vi "BC Async HP Data - SA.vi"(8 "error in (no error)":errorcluster, 11 "Bus Controller in":refnum<class "Bus Controller.lvclass">) -> (0 "error out":errorcluster, 3 "Bus Controller out":refnum<class "Bus Controller.lvclass">)   [LabVIEW 2020, in "Unit Tests.lvlib" / "Bus Controller.lvclass"]
uses:
  Bus Controller.lvclass
  Frames & Messages/TypeDefs/Async Message Config.ctl
  Frames & Messages/TypeDefs/Command Config.ctl
  Frames & Messages/TypeDefs/Command Type.ctl
  Frames & Messages/TypeDefs/Command Terminal Address.ctl
  Frames & Messages/TypeDefs/Command SubAddress.ctl
  Frames & Messages/TypeDefs/Command Word Count.ctl
  Frames & Messages/TypeDefs/Message Control.ctl
  Frames & Messages/TypeDefs/Simplified Parameter Data Table.ctl
  Frames & Messages/TypeDefs/Scaling Information.ctl
  Bus Controller.lvclass/Bus Controller.ctl
  1553 Session/1553 Session.lvclass/1553 Session.ctl
  Bus Controller/Bus Controller.lvclass
  1553 Component/1553 Component.lvclass/1553 Component.ctl
  <vilib>/addons/_JKI Toolkits/Caraya/classes/Assert/Assert True.vi
  1553 Component/1553 Component.lvclass
  1553 SubComponent/1553 SubComponent.lvclass
  Dependencies/FPGA Interface/FPGA Interface.lvclass
  <vilib>/addons/_JKI Toolkits/Caraya/classes/Test/Test.lvclass
  Frames & Messages/Async Message/Async Message.lvclass
  BCI-1553 API.lvlib
  1553 Session/1553 Session.lvclass
  <vilib>/addons/_JKI Toolkits/Caraya/classes/Assert/Assert.lvclass
panel:
  out "Data":u16[](array[numeric]) format="%04x"
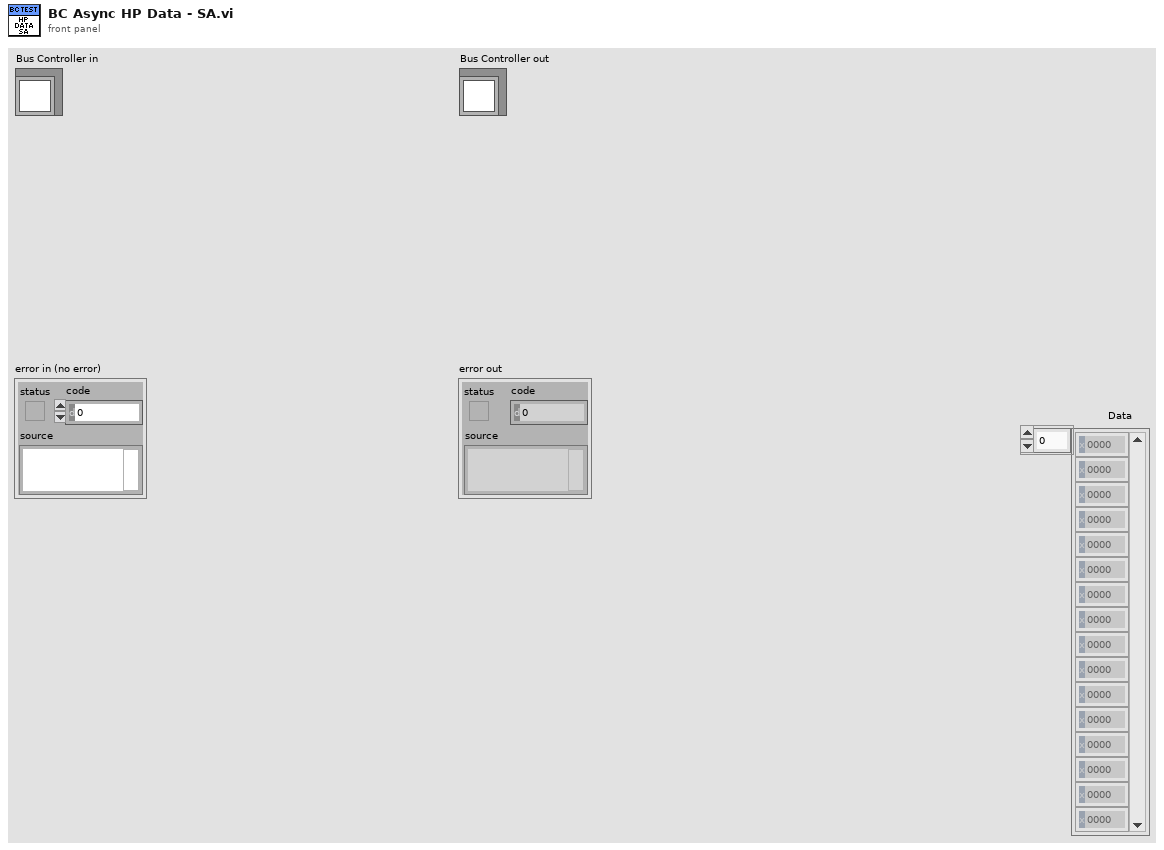
[diagram p1: front panel]
types:
  T1 = typedef "BCI-1553 API.lvlib/Command Word Count.ctl" = enum16{"1", "2", "3", "4", "5", "6", "7", "8", "9", "10", "11", "12", "13", "14", "15", "16", "17", "18", "19", "20", "21", "22", "23", "24", "25", "26", "27", "28", "29", "30", "31", "32"}
  T2 = typedef "BCI-1553 API.lvlib/Command SubAddress.ctl" = enum16{"Mode Code", "1", "2", "3", "4", "5", "6", "7", "8", "9", "10", "11", "12", "13", "14", "15", "16", "17", "18", "19", "20", "21", "22", "23", "24", "25", "26", "27", "28", "29", "30"}
  T3 = typedef "BCI-1553 API.lvlib/Command Terminal Address.ctl" = enum16{"0", "1", "2", "3", "4", "5", "6", "7", "8", "9", "10", "11", "12", "13", "14", "15", "16", "17", "18", "19", "20", "21", "22", "23", "24", "25", "26", "27", "28", "29", "30", "Broadcast"}
  T4 = typedef "BCI-1553 API.lvlib/Command Type.ctl" = enum16{"Transmit", "Receive"}
  T5 = typedef "BCI-1553 API.lvlib/Simplified Parameter Data Table.ctl" = cluster{"Parameter Name":string, "Base Word":u16, "Scaling Info":T6}
  T6 = typedef "BCI-1553 API.lvlib/Scaling Information.ctl" = cluster{"Bit Offset":i32, "Bit Count":i32, "LSB Resolution":dbl, "2's Complement":bool, "Big Endian":bool, "Sign Bit":bool}
  T7 = typedef "BCI-1553 API.lvlib/Command Config.ctl" = cluster{"Command Type":T4, "Terminal Address":T3, "SubAddress":T2, "Word Count\\Mode Code":T1, "Command Data":u16[]}
  T8 = typedef "BCI-1553 API.lvlib/Async Message Config.ctl" = cluster{"Group":i32, "High Priority":bool, "Time to Next Msg (100 us)":u16, "Command Config":T7, "Message Control":T9}
  T9 = typedef "BCI-1553 API.lvlib/Message Control.ctl" = cluster{"MC17 Time Sync":bool, "Error Mask":bool, "Service Request Mask":bool, "Busy Mask":bool, "SubSystem Flag Mask":bool, "Terminal Flag Mask":bool, "Reserved Mask":bool, "Retry":bool, "Bus A / !Bus B":bool, "Self-Test Loopback":bool, "Broadcast Mask":bool, "EoM Interrupt":bool, "Mode Code Format":bool, "Broadcast Format":bool, "RT-RT Format":bool}
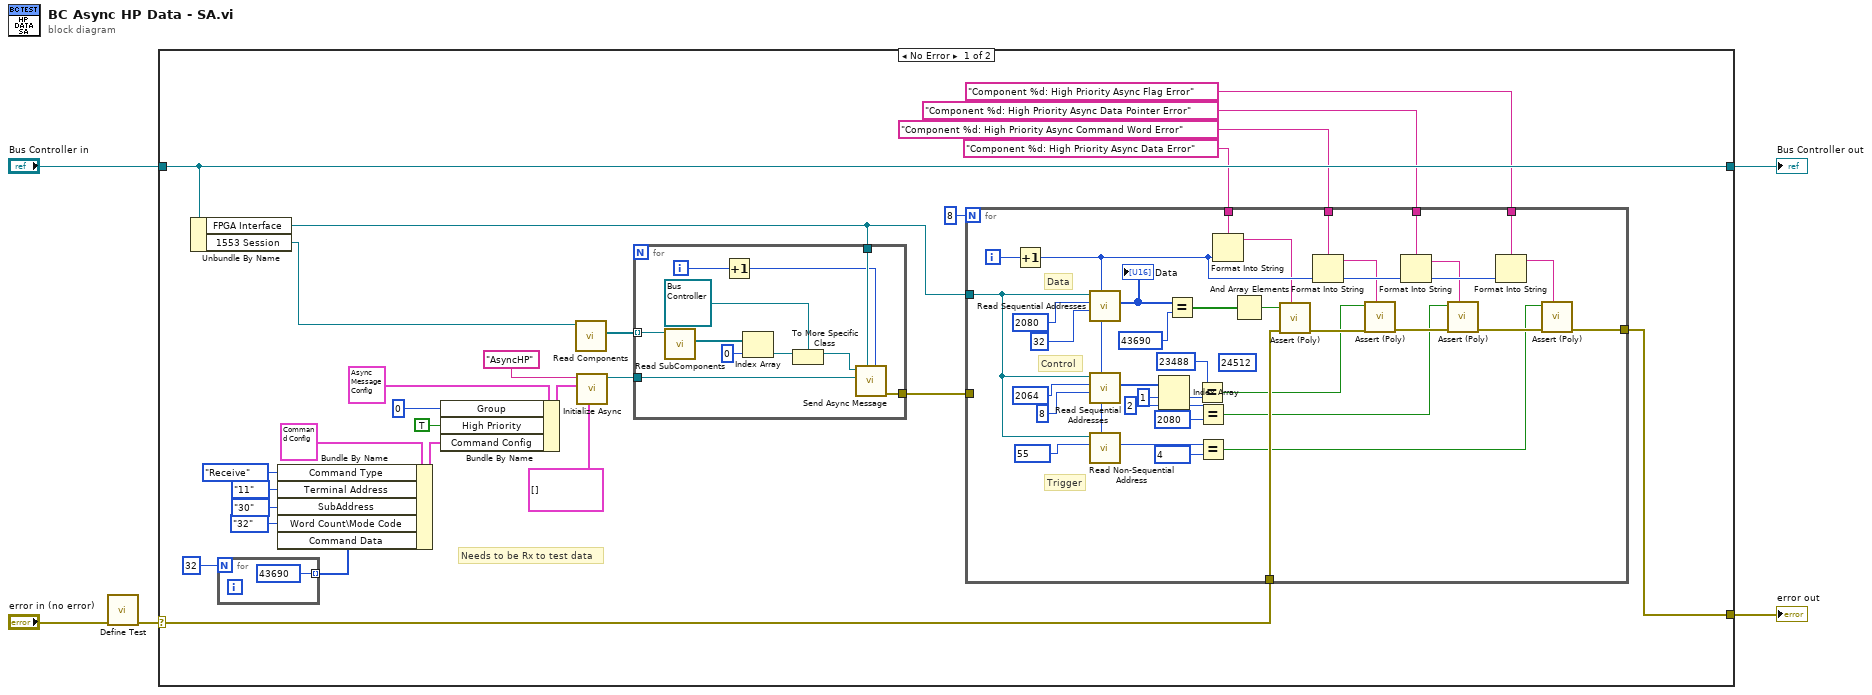
[diagram p0: block diagram]
diagram:
  n1 = call <vilib>:"Define Test.vi"("error in (no error)"="error in (no error)") -> ("error out"=w1:errorcluster)  [unwired: 9 in, 1 out]
  n2 = case shown="No Error" w1 {
    selector: w1 -> [w18 w83]
    tunnel: [w17 w83] -> w5
    tunnel: [w32 w82] -> w3
    tunnel: "Bus Controller in" -> [w32 w82]
    frame No Error {
      # "Needs to be Rx to test data"
      n3 = Unbundle By Name(w32) -> ("FPGA Interface"=w19:refnum<class "FPGA Interface.lvclass">, "1553 Session"=w22:refnum<class "1553 Session.lvclass">)
      n4 = for {
        N: 32 -> [_]
        tunnel: [u16 43690] -> w23 mode=indexing
      }
      n5 = Bundle By Name(cluster=T7 {"Command Type"=enum."Transmit", "Terminal Address"=enum."0", "SubAddress"=enum."Mode Code", "Word Count\\Mode Code"=enum."1", "Command Data"=[]} ("Command Config"), "Command Type"=Command_Type."Receive", "Terminal Address"=Command_Terminal_Address."11", "SubAddress"=Command_SubAddress."30", "Word Count\\Mode Code"=Command_Word_Count."32" ("Word Count\\Mode Code"), "Command Data"=w23) -> (w26:T7)
      n6 = Bundle By Name(cluster=T8 {"Group"=0, "High Priority"=FALSE, "Time to Next Msg (100 us)"=0, "Command Config"={"Command Type"=enum."Transmit", "Terminal Address"=enum."0", "SubAddress"=enum."Mode Code", "Word Count\\Mode Code"=enum."1", "Command Data"=[]}, "Message Control"={"MC17 Time Sync"=FALSE, "Error Mask"=FALSE, "Service Request Mask"=FALSE, "Busy Mask"=FALSE, "SubSystem Flag Mask"=FALSE, "Terminal Flag Mask"=FALSE, "Reserved Mask"=FALSE, "Retry"=FALSE, "Bus A / !Bus B"=FALSE, "Self-Test Loopback"=FALSE, "Broadcast Mask"=FALSE, "EoM Interrupt"=FALSE, "Mode Code Format"=FALSE, "Broadcast Format"=FALSE, "RT-RT Format"=FALSE}} ("Async Message Config"), "Group"=0, "High Priority"=TRUE, "Command Config"=w26) -> (w29:T8)
      n7 = call "Read Components.vi"("1553 Board in"=w22) -> ("Components"=w21:refnum<class "1553 Component.lvclass">[])  [unwired: 8 in, 2 out]
      n8 = call "Initialize Async.vi"("Parameters"=T5[] [], "Async Message Config"=w29, "ID"="AsyncHP") -> ("Async Message out"=w20:refnum<class "Async Message.lvclass">)  [unwired: 7 in, 1 out]
      n9 = for {
        tunnel: w21 -> [w80] mode=indexing
        tunnel: w20 -> [w74]
        tunnel: w19 -> [w73]
        tunnel: [w70] -> w6
        i -> [w72]
        n10 = call "Read SubComponents.vi"("1553 Component in"=w80) -> ("SubComponents"=w79:refnum<class "1553 SubComponent.lvclass">[])  [unwired: 8 in, 2 out]
        n11 = Increment(x=w72) -> (x+1=w71:i32)
        n12 = Index Array(array=w79, index=0) -> (element=w77:refnum<class "1553 SubComponent.lvclass">)
        n13 = To More Specific Class(target class=refnum<class "Bus Controller.lvclass"> refnum ("SLSC 1553 API.lvlib:Bus Controller.lvclass"), reference=w77) -> (specific class reference=w75:refnum<class "Bus Controller.lvclass">)  [unwired: 1 in, 1 out]
        n14 = call-dynamic "Send Async Message.vi"("Component ID"=w71, "FPGA Interface"=w73, "Async Message"=w74, "Bus Controller in"=w75) -> ("error out"=w70:errorcluster)  [unwired: 6 in, 1 out]
      }
      n15 = for {
        N: 8 -> [_]
        tunnel: w19 -> [w55]
        tunnel: w18 -> [w45]
        tunnel: [w34] -> w17
        tunnel: "Component %d: High Priority Async Data Error" ("custom report message (\"\")") -> [w68]
        tunnel: "Component %d: High Priority Async Command Word Error" ("custom report message (\"\")") -> [w53]
        tunnel: "Component %d: High Priority Async Data Pointer Error" ("custom report message (\"\")") -> [w52]
        tunnel: "Component %d: High Priority Async Flag Error" ("custom report message (\"\")") -> [w51]
        tunnel: w6 -> [_]
        i -> [w69]
        (unwired) u16 24512
        # "Data"
        # "Trigger"
        # "Control"
        n16 = Increment(x=w69) -> (x+1=w50:i32)
        n17 = call-dynamic "Read Sequential Addresses.vi"("Target IC (1-8)"=w50, "Addresses to Read"=u16 32, "Starting Address"=u16 2080, "FPGA Interface in"=w55) -> ("Data"=w63:u16[])  [unwired: 6 in, 1 out]
        "Data" <- w63
        n18 = call-dynamic "Read Sequential Addresses.vi"("Target IC (1-8)"=w50, "Addresses to Read"=u16 8, "Starting Address"=u16 2064, "FPGA Interface in"=w55) -> ("Data"=w60:u16[])  [unwired: 6 in, 1 out]
        n19 = call-dynamic "Read Non-Sequential Address.vi"("Target IC (1-8)"=w50, "Address"=u16 55, "FPGA Interface in"=w55) -> ("Data"=w47:u16)  [unwired: 7 in, 1 out]
        n20 = Index Array(array=w60, index #1=1 ("index"), index #2=2 ("index")) -> (element #1=w56:u16, element #2=w48:u16)
        n21 = Equal?(x=w63, y=u16 43690) -> (x = y?=w61:bool[])
        n22 = Equal?(x=u16 23488, y=w56) -> (x = y?=w41:bool)
        n23 = Equal?(x=w48, y=u16 2080) -> (x = y?=w39:bool)
        n24 = Equal?(x=w47, y=u16 4) -> (x = y?=w36:bool)
        n25 = Format Into String(format string=w68, w50) -> (resulting string=w44:string)  [unwired: 2 in, 1 out]
        n26 = And Array Elements(Boolean array=w61) -> (logical AND=w46:bool)
        n27 = call-poly <vilib>:"Assert (Poly).vi"("Label"=w44, "error in (no error)"=w45, "True?"=w46) -> ("error out"=w43:errorcluster)  [unwired: 7 in, 1 out]
        n28 = Format Into String(format string=w53, w50) -> (resulting string=w42:string)  [unwired: 2 in, 1 out]
        n29 = call-poly <vilib>:"Assert (Poly).vi"("Label"=w42, "error in (no error)"=w43, "True?"=w41) -> ("error out"=w40:errorcluster)  [unwired: 7 in, 1 out]
        n30 = Format Into String(format string=w52, w50) -> (resulting string=w38:string)  [unwired: 2 in, 1 out]
        n31 = call-poly <vilib>:"Assert (Poly).vi"("Label"=w38, "error in (no error)"=w40, "True?"=w39) -> ("error out"=w37:errorcluster)  [unwired: 7 in, 1 out]
        n32 = Format Into String(format string=w51, w50) -> (resulting string=w35:string)  [unwired: 2 in, 1 out]
        n33 = call-poly <vilib>:"Assert (Poly).vi"("Label"=w35, "error in (no error)"=w37, "True?"=w36) -> ("error out"=w34:errorcluster)  [unwired: 7 in, 1 out]
      }
    }
    frame Error {
    }
  }
  "error out" <- w5
  "Bus Controller out" <- w3
